vi "destroy.vi"(8 "error in (no error)":errorcluster, 11 "ComicVine_manager in":refnum<class "ComicVine_manager.lvclass">) -> (0 "error out":errorcluster)   [LabVIEW 2024, in "ComicVine_manager.lvclass"]
uses:
  ComicVine_manager.lvclass
  ComicVine_manager.lvclass/ComicVine_manager.ctl
  states--enum.ctl
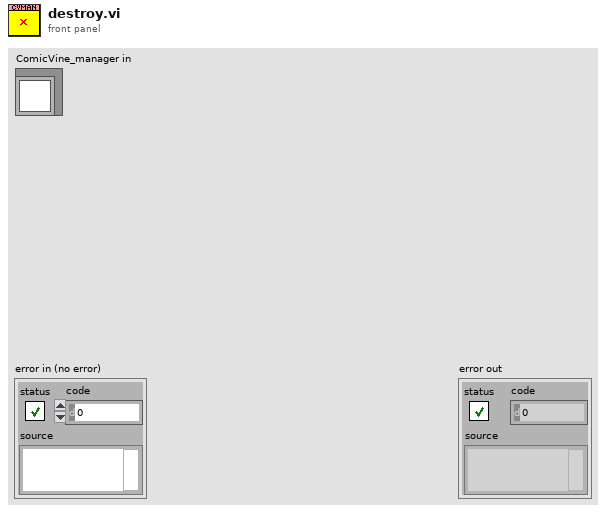
[diagram p1: front panel]
types:
  T1 = typedef "ComicVine_manager.lvclass/states--enum.ctl" = enum16{"start", "running", "start timer", "update file", "set directories", "wait", "shutdown"}
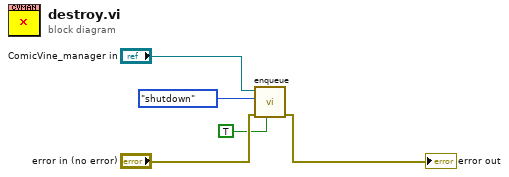
[diagram p0: block diagram]
diagram:
  n1 = call "enqueue.vi"("priority (f)"=TRUE, "error in (no error)"="error in (no error)", "cmd"=states--enum."shutdown", "ComicVine_manager in"="ComicVine_manager in") -> ("error out"=→"error out":errorcluster)  [unwired: 6 in, 1 out]
